vi "ReadStopEvent.vi"(8 "error in (no error)":errorcluster, 11 "object in":refnum<class "Logger.lvclass">) -> (0 "error out":errorcluster, 2 "StopEvent":refnum<user-event>, 3 "object out":refnum<class "Logger.lvclass">)   [LabVIEW 2014, in "Logger.lvclass"]
uses:
  Logger.lvclass
  Logger.lvclass/Logger.ctl
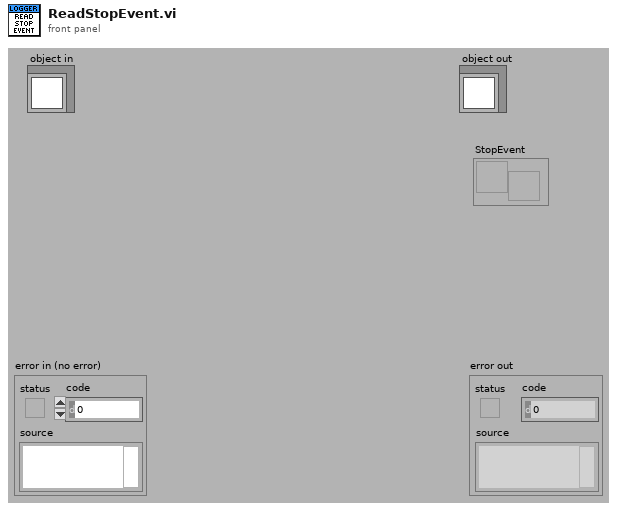
[diagram p1: front panel]
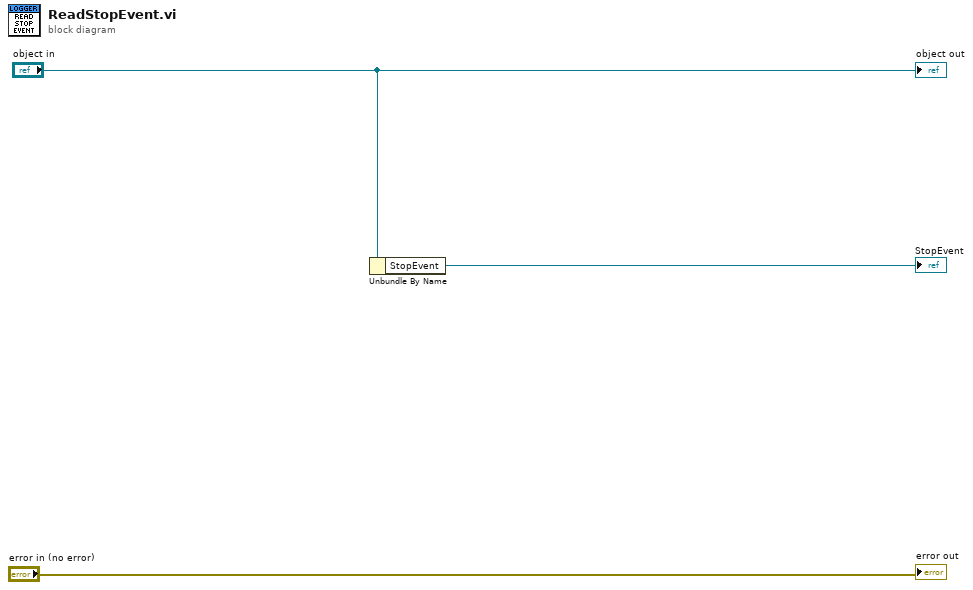
[diagram p0: block diagram]
diagram:
  n1 = Unbundle By Name("object in") -> ("StopEvent"=→"StopEvent":refnum<user-event>)
  "error out" <- "error in (no error)"
  "object out" <- "object in"
